vi "Write bandwidth.vi"(8 "error in (no error)":errorcluster, 10 "bandwidth":i16, 11 "Load New Speaker Chirp in":refnum<class "Load New Speaker Chirp.lvclass">) -> (0 "error out":errorcluster, 3 "Load New Speaker Chirp out":refnum<class "Load New Speaker Chirp.lvclass">)   [LabVIEW 2014, in "ePAS Library.lvlib" / "Load New Speaker Chirp.lvclass"]
uses:
  Load New Speaker Chirp.lvclass
  Load New Speaker Chirp.lvclass/Load New Speaker Chirp.ctl
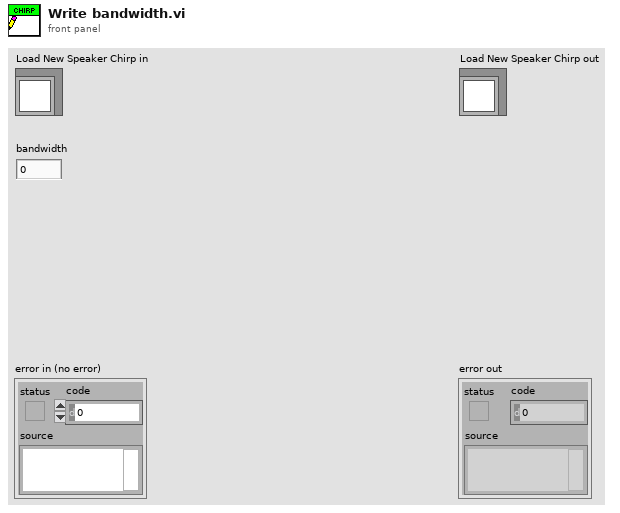
[diagram p1: front panel]
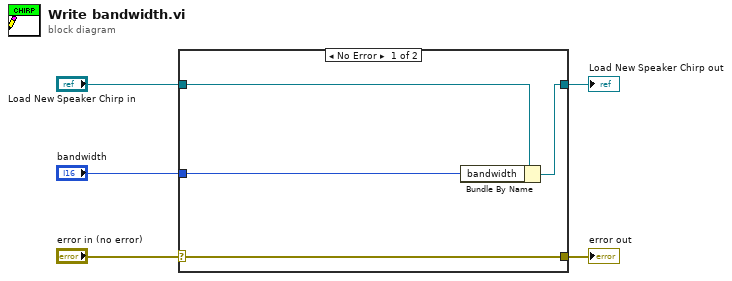
[diagram p0: block diagram]
diagram:
  n1 = case shown="No Error" "error in (no error)" {
    selector: "error in (no error)" -> [w9 w10]
    tunnel: [w9 w10] -> w4
    tunnel: [w7 w11] -> w2
    tunnel: "Load New Speaker Chirp in" -> [w8 w11]
    tunnel: "bandwidth" -> [w6 _]
    frame No Error {
      n2 = Bundle By Name(cluster=w8, "bandwidth"=w6) -> (w7:refnum<class "Load New Speaker Chirp.lvclass">)
    }
    frame Error {
    }
  }
  "error out" <- w4
  "Load New Speaker Chirp out" <- w2
